vi "Verify PS ComPorts.vi"(0 "Sequence path":path=path "C:/ModisEdge/Scanner/Test Sequence/ModisEdgeScanner.ini", 5 "file name":string="ModisEdgeScanner.ini", 11 "error in (no error)":errorcluster) -> (2 "PS1_COMPort":string, 13 "PS2_COMPort":string)   [LabVIEW 2015]
doc: "Use this template to build a VI to use as a subVI."
uses:
  <vilib>/Utility/config.llb/Read Key (String).vi
  <vilib>/Utility/config.llb/NI_LVConfig.lvlib
  <instrlib>/BK Precision 178XB Series/BK Precision 178XB Series.lvlib
  <instrlib>/Keithley 27XX/Keithley 27XX.lvlib
panel:
  in  "Serial Configuration":T1={"Baud Rate"=9600, "Parity"=0, "Data Bits"=8, "Stop Bits"=10} {"Stop Bits" items=["1.0"=10]; "Data Bits" items=["8"=8]; "Parity" items=["None", "Odd", "Even"]; "Baud Rate" items=["4800"=4800, "9600"=9600, "19200"=19200, "38400"=38400]}
  out "error IO":errorcluster
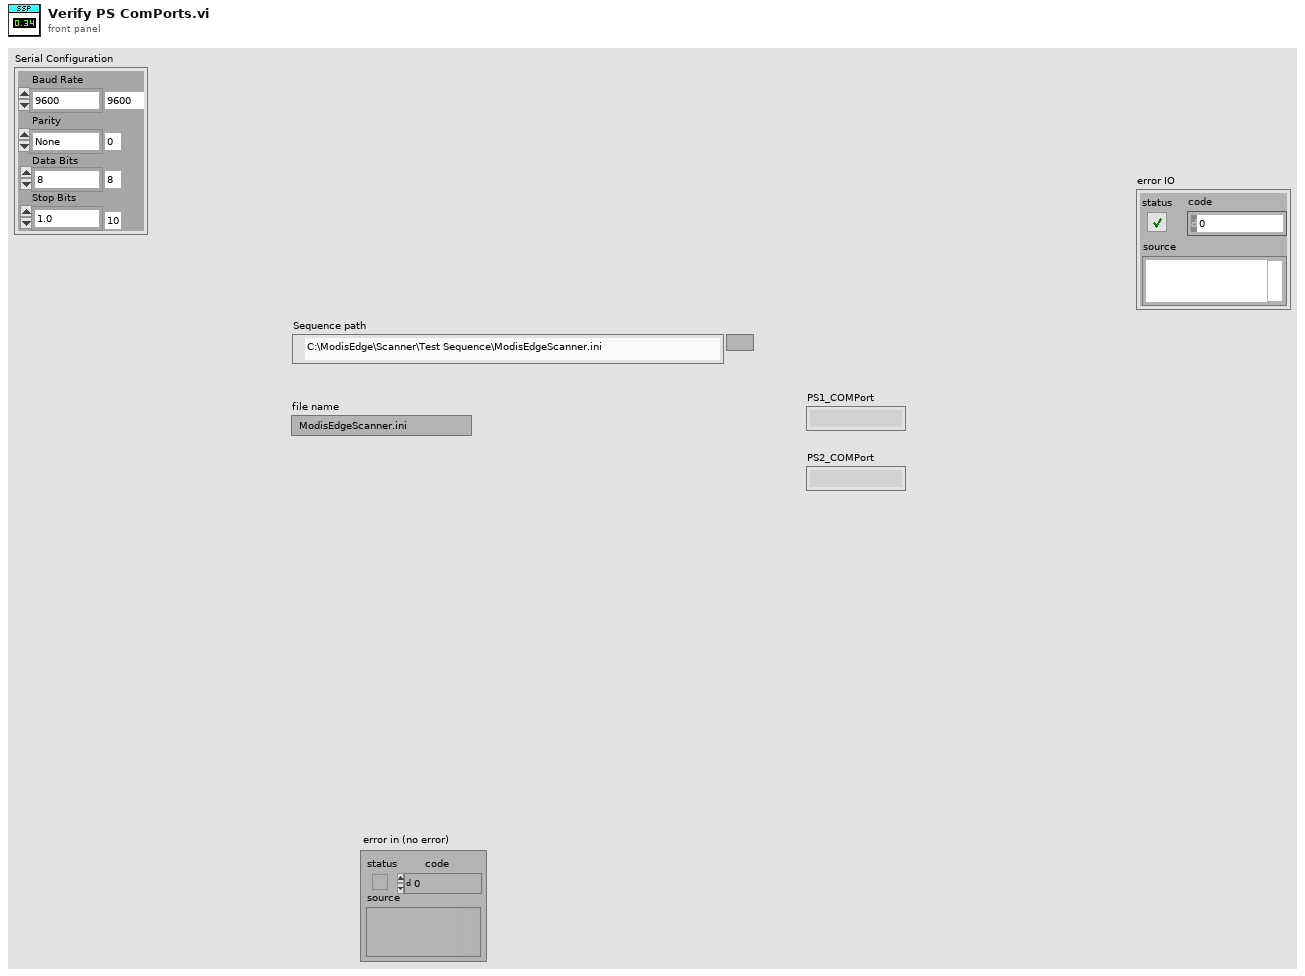
[diagram p1: front panel]
types:
  T1 = cluster{"Baud Rate":u32, "Parity":u16, "Data Bits":u16, "Stop Bits":u16}
  T2 = typedef "NI_LVConfig.lvlib/Config Data RefNum.ctl" = refnum<k1>
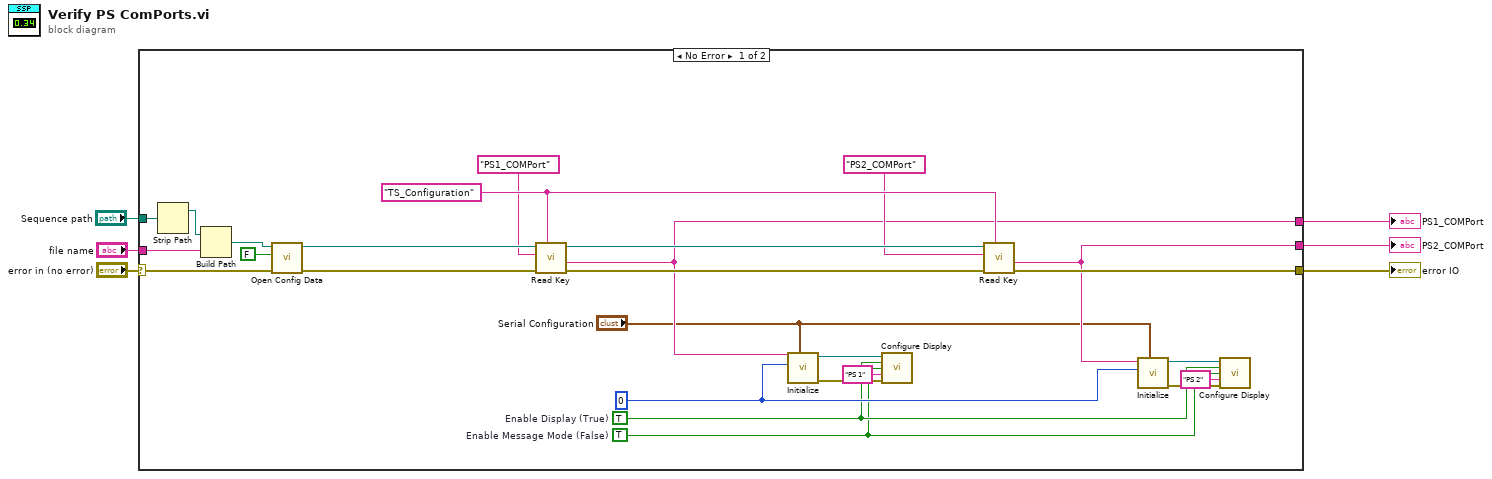
[diagram p0: block diagram]
diagram:
  n1 = case shown="No Error" "error in (no error)" {
    selector: "error in (no error)" -> [w32 w33]
    tunnel: [w19 w33] -> w1
    tunnel: "Sequence path" -> [w30 _]
    tunnel: "file name" -> [w28 _]
    tunnel: [w18 _] -> w3
    tunnel: [w17 _] -> w2
    frame No Error {
      w9 = TRUE  # Enable Message Mode (False)
      w10 = TRUE  # Enable Display (True)
      w15 = u8 0 ("Communication Address (0)")
      w24 = "TS_Configuration" ("key")
      n2 = Strip Path(path=w30) -> (stripped path=w29:path)  [unwired: 1 out]
      n3 = Build Path(base path=w29, name or relative path=w28) -> (appended path=w31:path)
      n4 = call <vilib>:"Open Config Data.vi"("error in (no error)"=w32, "create file if necessary (T)"=FALSE, "configuration file path"=w31) -> ("error out"=w26:errorcluster, "refnum"=w25:T2)  [unwired: 6 in, 1 out]
      n5 = call-poly <vilib>:"Read Key.vi"("section"=w24, "error in (no error)"=w26, "key"="PS1_COMPort", "refnum"=w25) -> ("error out"=w23:errorcluster, "value"=w18:string, "refnum out"=w22:T2)  [unwired: 4 in, 1 out]
      n6 = call <instrlib>:"Initialize.vi"("Serial Configuration"="Serial Configuration", "Communication Address (0)"=w15, "VISA resource name"=w18) -> ("error out"=w13:errorcluster, "VISA resource name out"=w14:refnum<visa-resource-name>)  [unwired: 7 in]
      n7 = call <instrlib>:"Configure Display.vi"("VISA resource name"=w14, "Enable Display (True)"=w10, "Enable Message Mode (False)"=w9, "Message (Empty)"="PS 1", "error in (no error)"=w13) -> ()  [unwired: 9 in, 2 out]
      n8 = call-poly <vilib>:"Read Key.vi"("section"=w24, "error in (no error)"=w23, "key"="PS2_COMPort", "refnum"=w22) -> ("error out"=w19:errorcluster, "value"=w17:string)  [unwired: 4 in, 2 out]
      n9 = call <instrlib>:"Initialize.vi"("Serial Configuration"="Serial Configuration", "Communication Address (0)"=w15, "VISA resource name"=w17) -> ("error out"=w12:errorcluster, "VISA resource name out"=w11:refnum<visa-resource-name>)  [unwired: 7 in]
      n10 = call <instrlib>:"Configure Display.vi"("VISA resource name"=w11, "Enable Display (True)"=w10, "Enable Message Mode (False)"=w9, "Message (Empty)"="PS 2", "error in (no error)"=w12) -> ()  [unwired: 9 in, 2 out]
    }
    frame Error {
    }
  }
  "PS1_COMPort" <- w3
  "PS2_COMPort" <- w2
  "error IO" <- w1
